vi "fftw_flags_to_u32.vi"(1 "FFTW flags":T1) -> (0 "FFTW flags combined":u32)   [LabVIEW 2020, in "FFTWDLL.lvlib"]
doc: "Combine FFTW flags to U32 number compatible with FFTW lib."
uses:
  FFTWDLL.lvlib
  fftw_const_flags.ctl
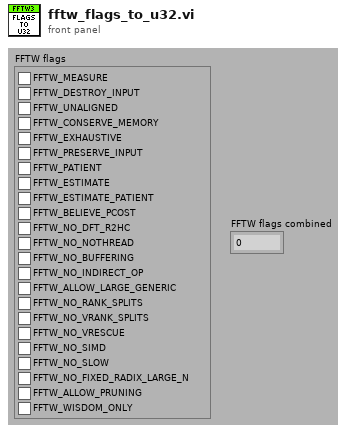
[diagram p1: front panel]
types:
  T1 = typedef "FFTWDLL.lvlib/fftw_const_flags.ctl" = cluster{"FFTW_MEASURE":bool, "FFTW_DESTROY_INPUT":bool, "FFTW_UNALIGNED":bool, "FFTW_CONSERVE_MEMORY":bool, "FFTW_EXHAUSTIVE":bool, "FFTW_PRESERVE_INPUT":bool, "FFTW_PATIENT":bool, "FFTW_ESTIMATE":bool, "FFTW_ESTIMATE_PATIENT":bool, "FFTW_BELIEVE_PCOST":bool, "FFTW_NO_DFT_R2HC":bool, "FFTW_NO_NOTHREAD":bool, "FFTW_NO_BUFFERING":bool, "FFTW_NO_INDIRECT_OP":bool, "FFTW_ALLOW_LARGE_GENERIC":bool, "FFTW_NO_RANK_SPLITS":bool, "FFTW_NO_VRANK_SPLITS":bool, "FFTW_NO_VRESCUE":bool, "FFTW_NO_SIMD":bool, "FFTW_NO_SLOW":bool, "FFTW_NO_FIXED_RADIX_LARGE_N":bool, "FFTW_ALLOW_PRUNING":bool, "FFTW_WISDOM_ONLY":bool}
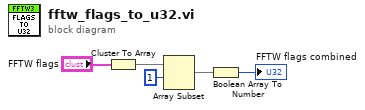
[diagram p0: block diagram]
diagram:
  n1 = Cluster To Array(cluster="FFTW flags") -> (array=w4:bool[])
  n2 = Array Subset(array=w4, index=1) -> (w2:bool[])  [unwired: 1 in]
  n3 = Boolean Array To Number(Boolean array=w2) -> (number=→"FFTW flags combined":u32)
